vi "check_connection.vi"(8 "error in (no error)":errorcluster caption="错误输入（无错误）", 11 "MotorSystem 输入":refnum<class "MotorSystem.lvclass">) -> (0 "error out":errorcluster caption="错误输出", 2 "changed?":bool, 3 "MotorSystem 输出":refnum<class "MotorSystem.lvclass">)   [LabVIEW 2016, in "MotionControl_UFO_3DOF.lvlib" / "MotorSystem.lvclass"]
uses:
  <userlib>/MotionControl_UFO_3DOF/MotorSystem/MotorSystem.lvclass
  <userlib>/MotionControl_UFO_3DOF/MotorSystem/MotorSystem.lvclass/MotorSystem.ctl
  <userlib>/MotionControl_UFO_3DOF/OneMotion/OneMotion.lvclass
  <userlib>/UISimCanFunc_wrapper/UISimCanFunc_wrapper.lvlib
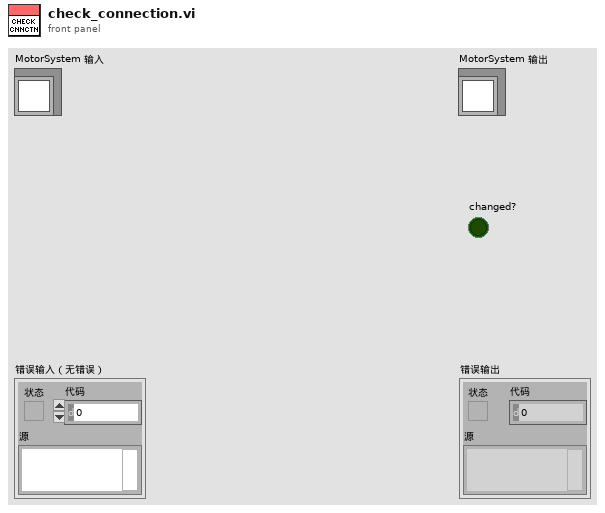
[diagram p1: front panel]
types:
  T1 = typedef "MotionControl_UFO_3DOF.lvlib/MotorSystem.lvclass/MotionCluster.ctl" = cluster{"OneMotion.lvclass":refnum<class "OneMotion.lvclass">, "connected?":bool, "default enabled?":bool, "enabled?":bool}
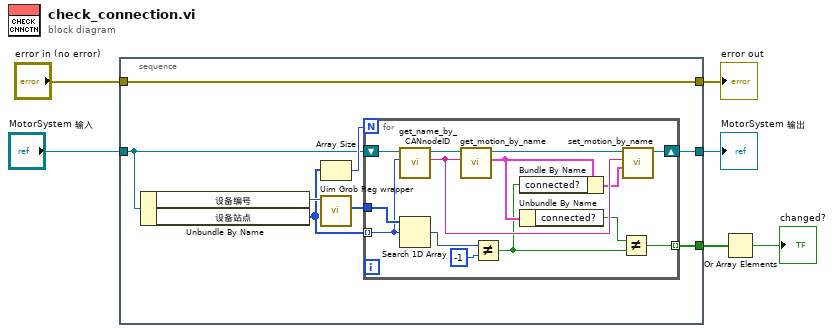
[diagram p0: block diagram]
diagram:
  n1 = stacked-sequence {
    tunnel: [w13] -> w6
    tunnel: [w8] -> w4
    tunnel: "MotorSystem 输入" -> [w9]
    tunnel: "error in (no error)" -> [w13]
    tunnel: [w7] -> w1
    frame #0 {
      n2 = Unbundle By Name(w9) -> ("设备编号"=w14:u32, "设备站点"=w11:u32[])
      n3 = Array Size(array=w11) -> (size(s)=w12:i32)
      n4 = call <userlib>:"Uim Grob Reg wrapper.vi"("dwDevIndex"=w14) -> ("pCanNodeIdList out"=w10:u32[])  [unwired: 8 in, 2 out]
      n5 = for {
        N: w12 -> [_]
        tunnel: w11 -> [w24] mode=indexing
        tunnel: w10 -> [w28]
        shift-right: [w19] -> w8
        shift-left: w9 -> [w25]
        tunnel: [w15] -> w7 mode=indexing
        n6 = call <userlib>:"get_name_by_CANnodeID.vi"("CAN node ID"=w24, "MotorSystem 输入"=w25) -> ("name"=w21:string, "MotorSystem 输出"=w23:refnum<class "MotorSystem.lvclass">)  [unwired: 6 in, 2 out]
        n7 = Search 1D Array(1D array=w28, element=w24) -> (index of element=w27:i32)  [unwired: 1 in]
        n8 = call <userlib>:"get_motion_by_name.vi"("name"=w21, "MotorSystem in"=w23) -> ("motion cluster"=w18:T1, "MotorSystem out"=w22:refnum<class "MotorSystem.lvclass">)  [unwired: 7 in, 1 out]
        n9 = Not Equal?(x=w27, y=-1) -> (x != y?=w16:bool)
        n10 = Bundle By Name(cluster=w18, "connected?"=w16) -> (w20:T1)
        n11 = Unbundle By Name(w18) -> ("connected?"=w17:bool)
        n12 = Not Equal?(x=w17, y=w16) -> (x != y?=w15:bool)
        n13 = call <userlib>:"set_motion_by_name.vi"("簇"=w20, "name"=w21, "MotorSystem输入"=w22) -> ("MotorSystem输出"=w19:refnum<class "MotorSystem.lvclass">)  [unwired: 7 in, 1 out]
      }
    }
  }
  "error out" <- w6
  "MotorSystem 输出" <- w4
  n14 = Or Array Elements(Boolean array=w1) -> (logical OR=→"changed?":bool)
